vi "Set RPC StreamOCVMeasurement __Output.vi"(7 "Streeming? (F)":bool, 8 "error in (no error)":errorcluster, 10 "Message Data":T1, 11 "gRPCid in":T2) -> (0 "error out":errorcluster)   [LabVIEW 2019, in "OCVServer.lvlib" / "OCVServer.lvclass"]
uses:
  OCVServer.lvclass
  gRPC lvSupport/Server API/typeDefs/grpcId.ctl
  RPC Messages/TemplateMessage/TemplateMessage_Data.ctl
  gRPC lvSupport/gprc-lvsupport.lvlib
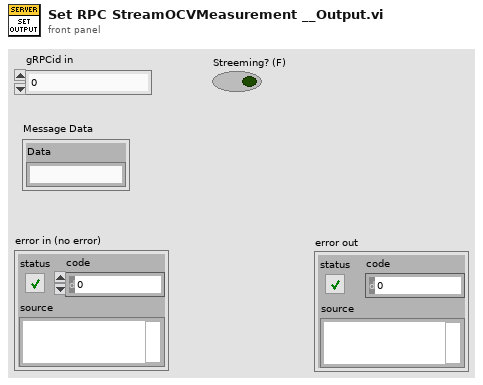
[diagram p1: front panel]
types:
  T1 = typedef "OCVServer.lvlib/OCVServer.lvclass/TemplateMessage_Data.ctl" = cluster{"Data":string}
  T2 = typedef "OCVServer.lvlib/gprc-lvsupport.lvlib/grpcId.ctl" = u64
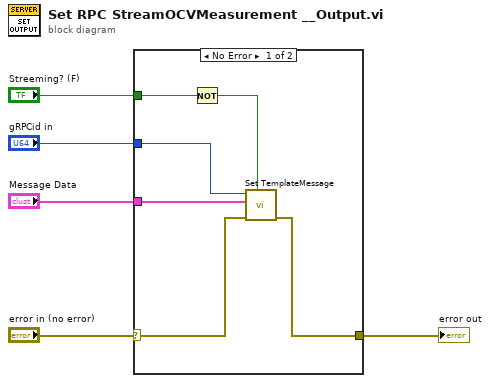
[diagram p0: block diagram]
diagram:
  n1 = case shown="No Error" "error in (no error)" {
    selector: "error in (no error)" -> [w11 w12]
    tunnel: [w9 w12] -> w4
    tunnel: "gRPCid in" -> [w10 _]
    tunnel: "Message Data" -> [w8 _]
    tunnel: "Streeming? (F)" -> [w7 _]
    frame No Error {
      n2 = Not(x=w7) -> (.not. x?=w6:bool)
      n3 = call "Set TemplateMessage.vi"("Complete Call (T)"=w6, "error in (no error)"=w11, "Message Data"=w8, "gRPCid"=w10) -> ("error out"=w9:errorcluster)  [unwired: 7 in]
    }
    frame Error {
    }
  }
  "error out" <- w4
